vi "AnglePidController (SubVI).vi"(4 "Sum Error":dbl, 5 "Previous Error":dbl, 6 "Wall Tracking Boolean":bool, 7 "Robot Width (m)":dbl, 10 "Desired Speed (m|s)":dbl, 11 "PID Setpoint [Wall Distance (m) OR Heading (deg)]":dbl) -> (0 "Velocity Right (m|s)":dbl, 1 "Sum For Shift Register":dbl, 2 "Current Error":dbl, 3 "Velocity Left (m|s)":dbl)   [LabVIEW 2017]
panel:
  in  "Angle D":dbl=0.0001
  in  "Angle I":dbl
  in  "Angle_P":dbl=0.002
  out "Angle Error":dbl(graph)
  out "Plot for Kd":dbl(graph)
  in  "kD":dbl=-0.1
  in  "kI":dbl
  in  "kP":dbl=0.12
  out "PID OUTPUT":dbl(graph)
  out "Current Error":dbl(graph)
  out "Shared Variable Heading (deg)":dbl
  out "Robot Heading (deg)":dbl
  in  "Right Encoder Distance (m)":dbl
  in  "Left Encoder Distance (m)":dbl
  # "VI Name: AnglePidController (SubVI).vi\nAuthor: Steven Lee\n\nThis SubVI takes in the Encoder Count values and provide PID control for the robot's heading.\n\nInput: Theta (Desired Angle), v0 (Desired Velocity)\nOutput: v_r (right wheel velocity), v_l (left wheel velocity)"
  # "Known working parameters\nP: 0.12\nI: 0\nD: -0.1"
  # "settle with the following parameters for now:\n\nP = 0.002\nI = 0\nD = 0.0001"
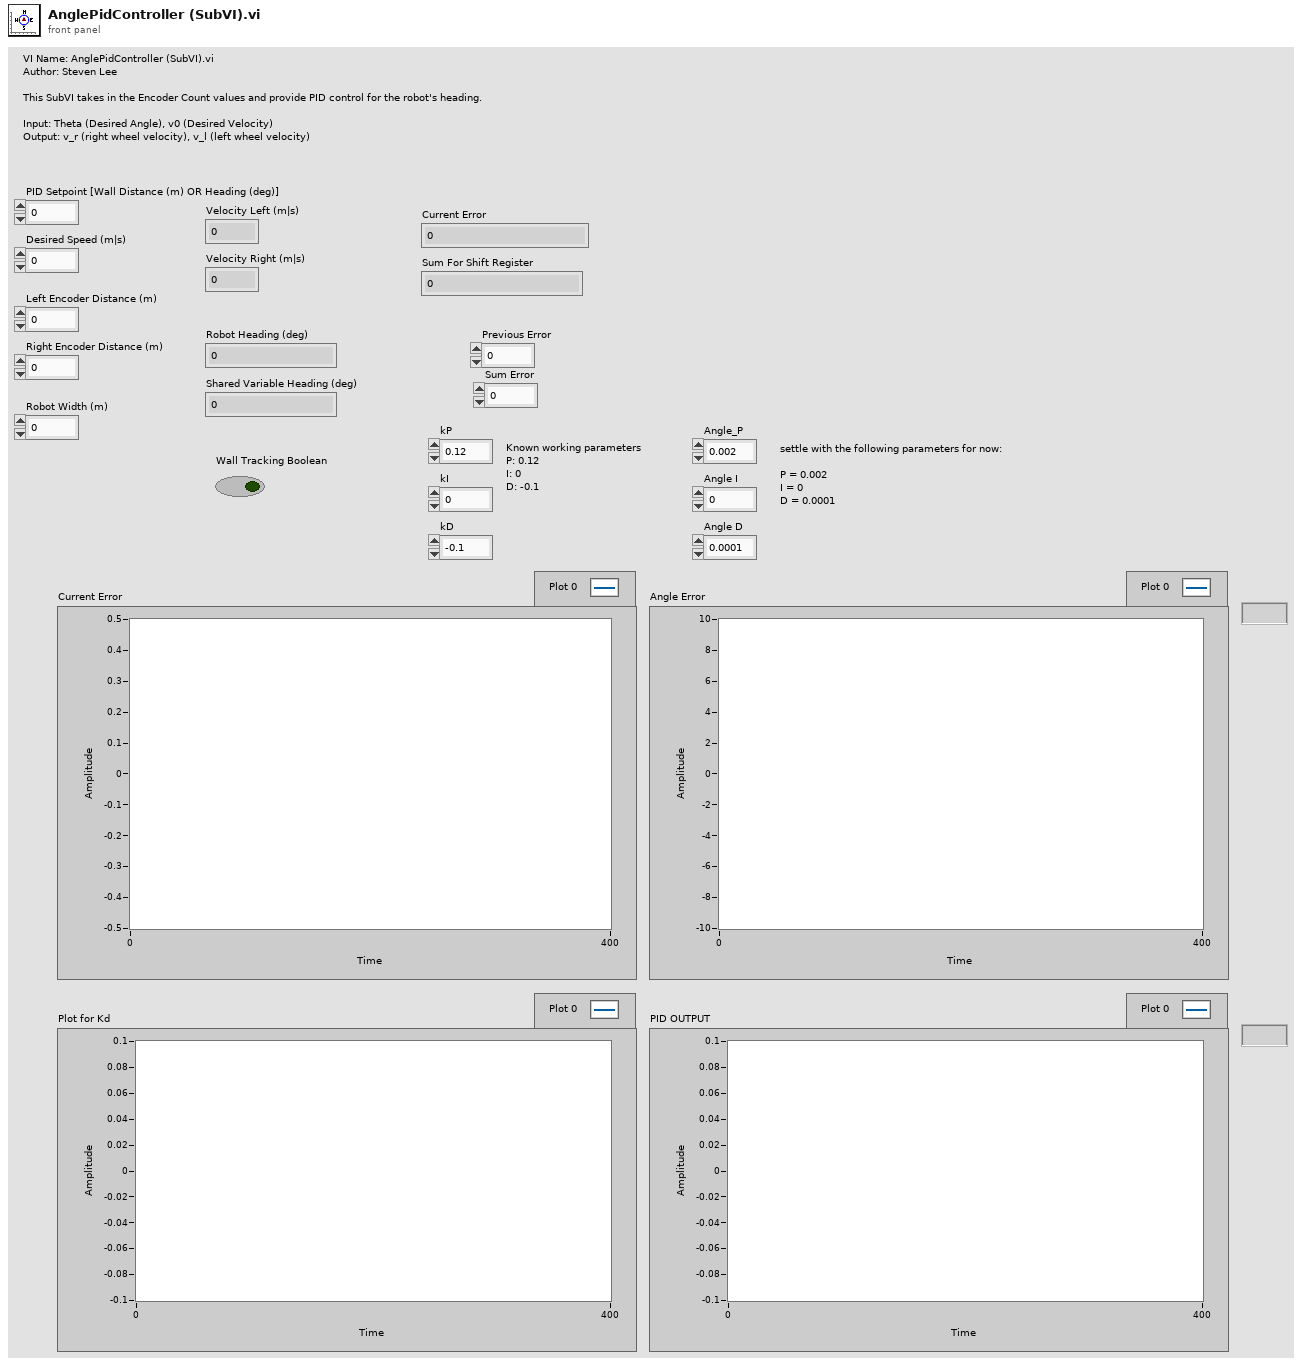
[diagram p1: front panel]
types:
  T1 = cluster{"proportional gain (Kc)":dbl, "integral time (Ti, min)":dbl, "derivative time (Td, min)":dbl}
  T2 = cluster{"Angle_P":dbl, "Angle I":dbl, "Angle D":dbl}
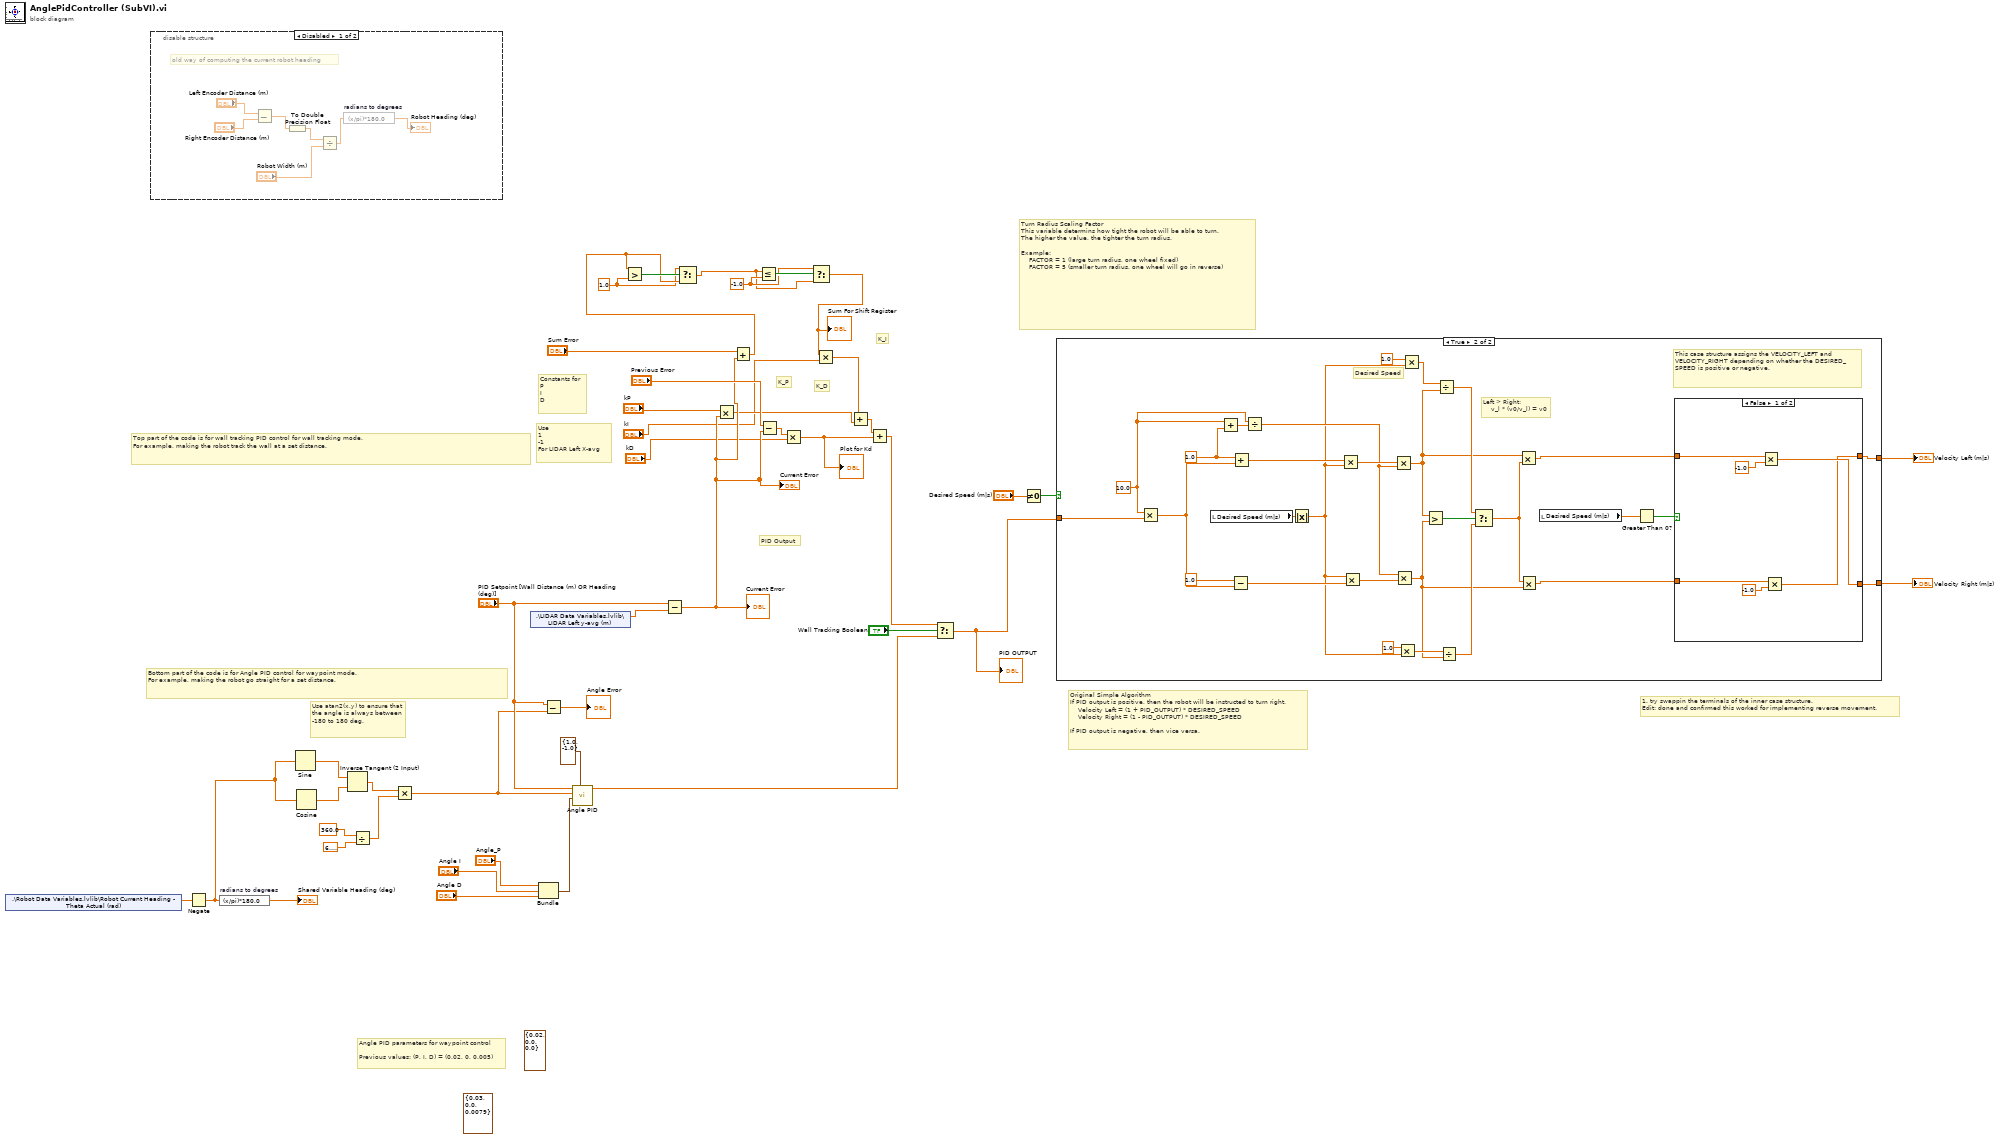
[diagram p0: block diagram]
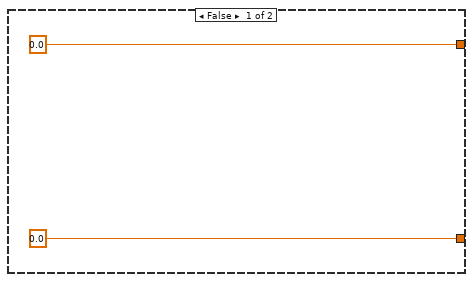
[diagram p3: hidden frame]
diagram:
  (unwired) T1 {"proportional gain (Kc)"=0.03, "integral time (Ti, min)"=0.0, "derivative time (Td, min)"=0.0079} ("PID gains")
  w25 = -1.0 ("y")
  w13 = 1.0 ("y")
  (unwired) T1 {"proportional gain (Kc)"=0.02, "integral time (Ti, min)"=0.0, "derivative time (Td, min)"=0.0} ("PID gains")
  # "Top part of the code is for wall tracking PID control for wall tracking mode.\nFor example, making the robot track the wall at a set distance."
  # "Bottom part of the code is for Angle PID control for waypoint mode.\nFor example, making the robot go straight for a set distance."
  # "K_I"
  # "K_P"
  # "K_D"
  # "Constants for\nP\nI\nD"
  # "Angle PID parameters for waypoint control\n\nPrevious values: (P, I, D) = (0.02, 0, 0.005)"
  # "Use atan2(x,y) to ensure that the angle is always between -180 to 180 deg."
  # "Use \n1\n-1\nFor LIDAR Left X-avg"
  # "Turn Radius Scaling Factor\nThis variable determins how tight the robot will be able to turn.\nThe higher the value, the tighter the turn radius.\n\nExample:\n    FACTOR = 1 (large turn radius, one wheel fixed)\n    FACTOR = 5 (smaller turn radius, one wheel will go in reverse)"
  # "1. try swappin the terminals of the inner case structure.\nEdit: done and confirmed this worked for implementing reverse movement."
  # "Original Simple Algorithm\nIf PID output is positive, then the robot will be instructed to turn right.\n    Velocity Left = (1 + PID_OUTPUT) * DESIRED_SPEED\n    Velocity Right = (1 - PID_OUTPUT) * DESIRED_SPEED\n\nIf PID output is negative, then vice versa."
  # "PID Output"
  n1 = shared-variable ".\\Robot Data Variables.lvlib\\Robot Current Heading - Theta Actual (rad)"() -> (w33:dbl)  [unwired: 1 in, 1 out]
  n2 = disable-structure shown="Disabled" {
    frame Disabled {
      # "old way of computing the current robot heading"
      n3 = Subtract(x="Left Encoder Distance (m)", y="Right Encoder Distance (m)") -> (x-y=w51:dbl)
      n4 = To Double Precision Float(number=w51) -> (double precision float=w50:dbl)
      n5 = Divide(x=w50, y="Robot Width (m)") -> (x/y=w45:dbl)
      n6 = expression code="(x/pi)*180.0" "radians to degrees"(w45) -> (→"Robot Heading (deg)":dbl)
    }
    frame Enabled {
    }
  }
  n7 = Negate(x=w33) -> (-x=w31:dbl)
  n8 = expression code="(x/pi)*180.0" "radians to degrees"(w31) -> (→"Shared Variable Heading (deg)":dbl)
  n9 = Sine(x=w31) -> (sin(x)=w39:dbl)
  n10 = Cosine(x=w31) -> (cos(x)=w38:dbl)
  n11 = Inverse Tangent (2 Input)(1:w38, 2:w39) -> (0:w36:dbl)
  n12 = Divide(x=360.0 ("y"), y=6.283185307179586) -> (x/y=w35:dbl)
  n13 = Multiply(x=w36, y=w35) -> (x*y=w6:dbl)
  n14 = shared-variable ".\\LIDAR Data Variables.lvlib\\LIDAR Left y-avg (m)"() -> (w12:dbl)  [unwired: 1 in, 1 out]
  n15 = Bundle("Angle_P"="Angle_P", "Angle I"="Angle I", "Angle D"="Angle D") -> (w1:T2)  [unwired: 1 in]
  n16 = Subtract(x="PID Setpoint [Wall Distance (m) OR Heading (deg)]", y=w6) -> (x-y=→"Angle Error":dbl)
  n17 = call "Angle PID.vi"("output range"=cluster{"output high":dbl, "output low":dbl} {"output high"=1.0, "output low"=-1.0}, "PID gains"=w1, "process variable"=w6, "setpoint"="PID Setpoint [Wall Distance (m) OR Heading (deg)]") -> ("output"=w9:dbl)  [unwired: 6 in, 1 out]
  n18 = Subtract(x="PID Setpoint [Wall Distance (m) OR Heading (deg)]", y=w12) -> (x-y=w28:dbl)
  "Current Error" <- w28
  "Current Error" <- w28
  n19 = Multiply(x="kP", y=w28) -> (x*y=w19:dbl)
  n20 = Add(x="Sum Error", y=w28) -> (x+y=w22:dbl)
  n21 = Greater?(x=w22, y=w13) -> (0:w27:bool)
  n22 = Select(t=w13, s=w27, f=w22) -> (s? t:f=w24:dbl)
  n23 = Less Or Equal?(x=w24, y=w25) -> (x <= y?=w26:bool)
  n24 = Subtract(x="Previous Error", y=w28) -> (x-y=w29:dbl)
  n25 = Multiply(x=w29, y="kD") -> (x*y=w14:dbl)
  "Plot for Kd" <- w14
  n26 = Select(t=w25, s=w26, f=w24) -> (s? t:f=w21:dbl)
  "Sum For Shift Register" <- w21
  n27 = Multiply(x=w21, y="kI") -> (x*y=w18:dbl)
  n28 = Add(x=w18, y=w19) -> (x+y=w20:dbl)
  n29 = Add(x=w20, y=w14) -> (x+y=w10:dbl)
  n30 = Select(t=w10, s="Wall Tracking Boolean", f=w9) -> (s? t:f=w8:dbl)
  "PID OUTPUT" <- w8
  n31 = Not Equal To 0?(x="Desired Speed (m|s)") -> (x != 0?=w40:bool)
  n32 = case shown="True" w40 {
    tunnel: w8 -> [_ w67]
    tunnel: [0.0 w55] -> w43
    tunnel: [0.0 w54] -> w42
    frame False {
    }
    frame True {
      w63 = 10.0 ("x")
      w65 = 1.0 ("x")
      # "This case structure assigns the VELOCITY_LEFT and VELOCITY_RIGHT depending on whether the DESIRED_SPEED is positive or negative."
      # "Desired Speed"
      # "Left > Right: \n    v_l * (v0/v_l) = v0"
      n33 = Multiply(x=w63, y=w67) -> (x*y=w66:dbl)
      n34 = local read "Desired Speed (m|s)"() -> (w61:dbl)
      n35 = Add(x=w63, y=w65) -> (x+y=w64:dbl)
      n36 = Subtract(x=1.0, y=w66) -> (x-y=w80:dbl)
      n37 = Add(x=w65, y=w66) -> (x+y=w81:dbl)
      n38 = Divide(x=w63, y=w64) -> (x/y=w62:dbl)
      n39 = Absolute Value(x=w61) -> (abs(x)=w60:dbl)
      n40 = Multiply(x=w81, y=w60) -> (x*y=w79:dbl)
      n41 = Multiply(x=w60, y=w80) -> (x*y=w78:dbl)
      n42 = Multiply(x=w79, y=w62) -> (x*y=w70:dbl)
      n43 = Multiply(x=w62, y=w78) -> (x*y=w69:dbl)
      n44 = Multiply(x=1.0, y=w60) -> (x*y=w73:dbl)
      n45 = Multiply(x=1.0, y=w60) -> (x*y=w75:dbl)
      n46 = Greater?(x=w70, y=w69) -> (0:w77:bool)
      n47 = Divide(x=w75, y=w70) -> (x/y=w72:dbl)
      n48 = Divide(x=w73, y=w69) -> (x/y=w71:dbl)
      n49 = Select(t=w72, s=w77, f=w71) -> (s? t:f=w68:dbl)
      n50 = Multiply(x=w70, y=w68) -> (x*y=w57:dbl)
      n51 = Multiply(x=w68, y=w69) -> (x*y=w56:dbl)
      n52 = local read "Desired Speed (m|s)"() -> (w58:dbl)
      n53 = Greater Than 0?(x=w58) -> (x > 0?=w59:bool)
      n54 = case shown="False" w59 {
        tunnel: w57 -> [w86 w90]
        tunnel: [w83 w90] -> w55
        tunnel: w56 -> [w85 w89]
        tunnel: [w84 w89] -> w54
        frame False {
          n55 = Multiply(x=w86, y=-1.0) -> (x*y=w84:dbl)
          n56 = Multiply(x=w85, y=-1.0) -> (x*y=w83:dbl)
        }
        frame True {
        }
      }
    }
  }
  "Velocity Left (m|s)" <- w43
  "Velocity Right (m|s)" <- w42
